vi "ge_GXMLGenerator.vi"(5 "Version String":string, 6 "String ID":string, 7 "Version Tag Name":string, 8 "error in":errorcluster, 10 "Variant":variant) -> (0 "error out":errorcluster, 2 "XML String Out":string)   [LabVIEW 2018]
doc: "Using a custom XML schema, this VI converts LabVIEW data into an XML string. Data elements within any compound structure (such as multidimensional arrays, sub-clusters, or arrays of clusters) are represented with an appropriate hierarchy. The name of each LabVIEW control directly maps to the name of each XML element.\n\nEach control name must begin with a letter and adhere to XML specifications. No two controls of the same hierarchy may have the same name. Supported datatypes include integer, floating, complex, enum, boolean, string, path, and timestamp."
uses:
  <vilib>/NI/GXML/_subVIs/GXML Generator/Main Rcrsv/Recursive Flatten.vi
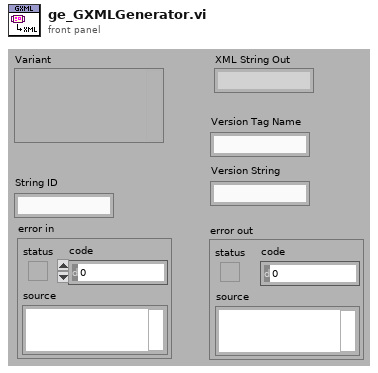
[diagram p1: front panel]
types:
  T1 = cluster{"In Empty Array?":bool, "Whitespace In":string}
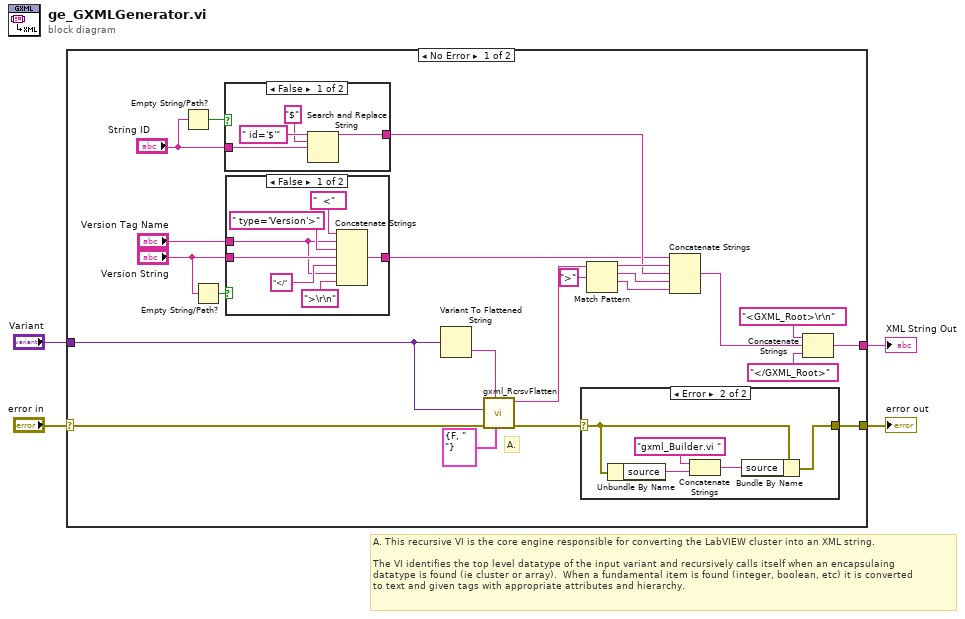
[diagram p0: block diagram]
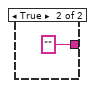
[diagram p2: hidden frame]
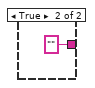
[diagram p3: hidden frame]
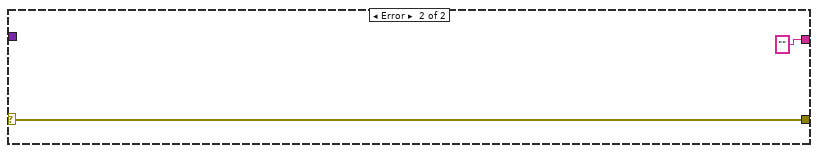
[diagram p5: hidden frame]
diagram:
  # "A. This recursive VI is the core engine responsible for converting the LabVIEW cluster into an XML string.  \n\nThe VI identifies the top level datatype of the input variant and recursively calls itself when an encapsulaing \ndatatype is found (ie cluster or array).  When a fundamental item is found (integer, boolean, etc) it is converted\nto text and given tags with appropriate attributes and hierarchy."
  n1 = case shown="No Error" "error in" {
    selector: "error in" -> [w23 w47]
    tunnel: [w21 "" ("XML String Out")] -> w4
    tunnel: "Variant" -> [w26 _]
    tunnel: [w24 w47] -> w2
    frame No Error {
      # "A."
      n2 = Empty String/Path?(string/path="String ID") -> (empty?=w9:bool)
      n3 = Empty String/Path?(string/path="Version String") -> (empty?=w18:bool)
      n4 = case shown="False" w9 {
        tunnel: "String ID" -> [w28 _]
        tunnel: [w27 ""] -> w12
        frame False {
          n5 = Search and Replace String(input string=" id='$'" ("string"), search string="$", replace string=w28) -> (result string=w27:string)  [unwired: 5 in, 3 out]
        }
        frame True {
        }
      }
      n6 = case shown="False" w18 {
        tunnel: "Version String" -> [w36 _]
        tunnel: "Version Tag Name" -> [w34 _]
        tunnel: [w32 ""] -> w5
        frame False {
          n7 = Concatenate Strings("  <" ("string"), w34, " type='Version'>" ("string"), w36, "</" ("string"), w34, ">\r\n" ("string")) -> (w32:string)
        }
        frame True {
        }
      }
      n8 = Variant To Flattened String(Variant=w26) -> (data string=w22:string)  [unwired: 1 out]
      n9 = call <vilib>:"gxml_RcrsvFlatten.vi"("HierarchyInfo"=T1 {"In Empty Array?"=FALSE, "Whitespace In"="  "}, "FlattenedData"=w22, "error in"=w23, "Variant"=w26) -> ("error out"=w25:errorcluster, "XML String Out"=w11:string)  [unwired: 5 in, 1 out]
      n10 = case shown="Error" w25 {
        selector: w25 -> [w40 w42]
        tunnel: [w40 w41] -> w24
        frame No Error {
        }
        frame Error {
          n11 = Unbundle By Name(w42) -> ("source"=w45:string)
          n12 = Concatenate Strings("gxml_Builder.vi ", w45) -> (w43:string)
          n13 = Bundle By Name(cluster=w42, "source"=w43) -> (w41:errorcluster)
        }
      }
      n14 = Match Pattern(string=w11, regular expression=">") -> (before substring=w13:string, match substring=w7:string, after substring=w6:string)  [unwired: 1 in, 1 out]
      n15 = Concatenate Strings(w5, w13, w12, w7, w6) -> (w10:string)
      n16 = Concatenate Strings("<GXML_Root>\r\n" ("string"), w10, "</GXML_Root>" ("string")) -> (w21:string)
    }
    frame Error {
    }
  }
  "XML String Out" <- w4
  "error out" <- w2
